vi "helloworld_serial.vi"() -> ()   [LabVIEW 2018]
uses:
  <vilib>/Instr/_visa.llb/VISA Configure Serial Port (Instr).vi
panel:
  in  "버퍼 쓰기":string
  in  "대기 시간 (ms)":u32
  out "에러 출력":errorcluster
  out "버퍼 읽기":string
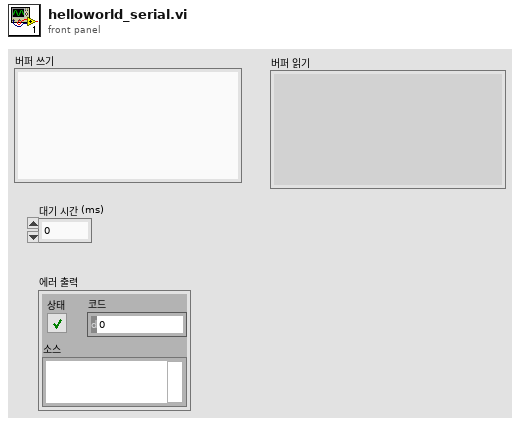
[diagram p1: front panel]
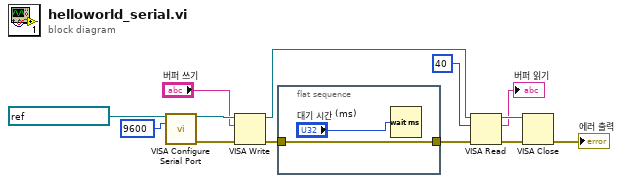
[diagram p0: block diagram]
diagram:
  n1 = call-poly "VISA Configure Serial Port"("VISA resource name"=refnum<visa-resource-name> "ASRL2::INSTR", "baud rate (9600)"=u32 9600) -> ("VISA resource name out"=w11:refnum<visa-resource-name>, "error out"=w10:errorcluster)  [unwired: 12 in]
  n2 = VISA Write(VISA resource name=w11, write buffer="버퍼 쓰기", error in (no error)=w10) -> (VISA resource name out=w6:refnum<visa-resource-name>, error out=w8:errorcluster)  [unwired: 1 out]
  n3 = flat-sequence {
    tunnel: w8 -> [w14]
    tunnel: [w14] -> w7
    frame #0 {
      n4 = Wait (ms)(milliseconds to wait="대기 시간 (ms)") -> ()  [unwired: 1 out]
    }
  }
  n5 = VISA Read(VISA resource name=w6, byte count=u32 40 ("바이트 카운트"), error in (no error)=w7) -> (VISA resource name out=w4:refnum<visa-resource-name>, read buffer=→"버퍼 읽기":string, error out=w3:errorcluster)  [unwired: 1 out]
  n6 = VISA Close(VISA resource name=w4, error in (no error)=w3) -> (error out=→"에러 출력":errorcluster)
